vi "Data Read Multiple.vi"(0 "VISA resource name":refnum<visa-resource-name>, 1 "Source (0: Function)":u16(ring) items=["Function", "Calculation 1"], 2 "Format (0: ASCII)":u16(ring) items=["ASCII", "Single Precision", "Double Precision"], 3 "Number of Readings (100)":i32=100, 4 "Sample Count (1)":i32=1, 5 "error in (no error)":errorcluster, 8 "Timeout (25000 ms)":u32=25000) -> (14 "VISA resource name out":refnum<visa-resource-name>, 15 "Data":dbl[](array[numeric]), 16 "Channels":i32[](array[numeric]), 17 "Units":string[](array[string]), 19 "error out":errorcluster)   [LabVIEW 2016, in "Keithley 2000.lvlib"]
doc: "This VI reads multiple measurements or calculations from the instrument. This VI should be used instead of the Data Read Single VI when you plan on reading many measurements at once or when you are reading measurements from many channels."
uses:
  Keithley 2000.lvlib
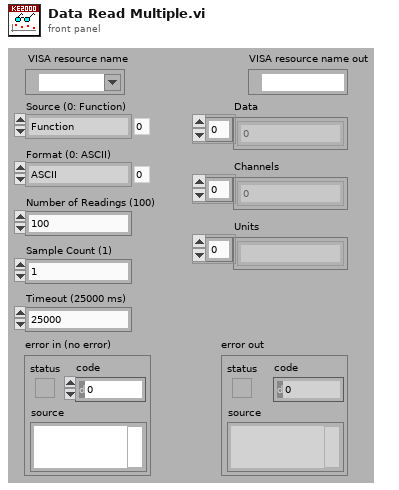
[diagram p1: front panel]
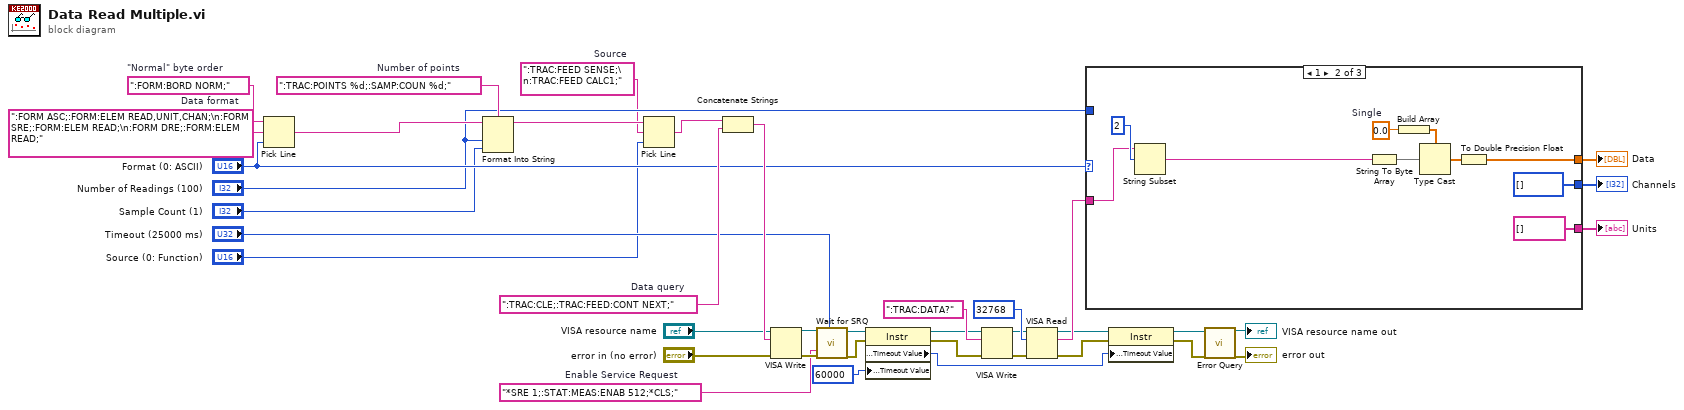
[diagram p0: block diagram]
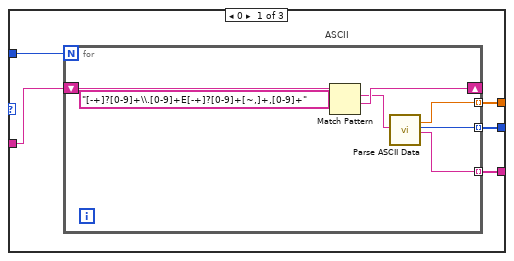
[diagram p2: hidden frame]
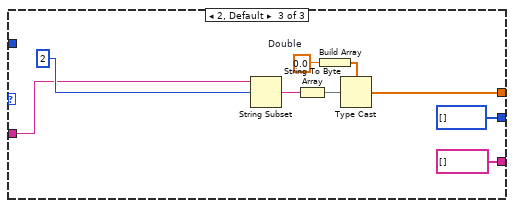
[diagram p3: hidden frame]
diagram:
  w19 = ":TRAC:FEED SENSE;\n:TRAC:FEED CALC1;"  # Source
  w1 = "*SRE 1;:STAT:MEAS:ENAB 512;*CLS;"  # Enable Service Request
  w36 = ":TRAC:POINTS %d;:SAMP:COUN %d;"  # Number of points
  w37 = ":FORM:BORD NORM;"  # "Normal" byte order
  w38 = ":FORM ASC;:FORM:ELEM READ,UNIT,CHAN;\n:FORM SRE;:FORM:ELEM READ;\n:FORM DRE;:FORM:ELEM READ;"  # Data format
  w34 = ":TRAC:CLE;:TRAC:FEED:CONT NEXT;"  # Data query
  n1 = Pick Line(string ("")=w37, multi-line string=w38, line index="Format (0: ASCII)") -> (output string=w35:string)
  n2 = Format Into String(format string=w36, initial string=w35, "Number of Readings (100)", "Sample Count (1)") -> (resulting string=w22:string)  [unwired: 1 in, 1 out]
  n3 = Pick Line(string ("")=w22, multi-line string=w19, line index="Source (0: Function)") -> (output string=w20:string)
  n4 = Concatenate Strings(w20, w34) -> (w33:string)
  n5 = VISA Write(VISA resource name="VISA resource name", write buffer=w33, error in (no error)="error in (no error)") -> (VISA resource name out=w28:refnum<visa-resource-name>, error out=w29:errorcluster)  [unwired: 1 out]
  n6 = call "Wait for SRQ.vi"("VISA resource name"=w28, "SRQ Enable Command"=w1, "error in (no error)"=w29, "Timeout (25000 ms)"="Timeout (25000 ms)") -> ("VISA resource name out"=w15:refnum<visa-resource-name>, "error out"=w14:errorcluster)  [unwired: 14 in]
  n7 = property class="Instr"(reference=w15, error in=w14, "General Settings:Timeout Value"=u32 60000) -> (reference out=w12:refnum<visa-resource-name>, error out=w11:errorcluster, "General Settings:Timeout Value"=w10:u32)
  n8 = VISA Write(VISA resource name=w12, write buffer=":TRAC:DATA?", error in (no error)=w11) -> (VISA resource name out=w17:refnum<visa-resource-name>, error out=w18:errorcluster)  [unwired: 1 out]
  n9 = VISA Read(VISA resource name=w17, byte count=u32 32768, error in (no error)=w18) -> (VISA resource name out=w9:refnum<visa-resource-name>, read buffer=w31:string, error out=w8:errorcluster)  [unwired: 1 out]
  n10 = case shown="1" "Format (0: ASCII)" {
    tunnel: [w43 w58 w64] -> w30
    tunnel: w31 -> [w44 w56 w66]
    tunnel: [w42 string[] [] string[] []] -> w26
    tunnel: [w41 i32[] [] i32[] []] -> w25
    tunnel: "Number of Readings (100)" -> [w40 _ _]
    frame 0 {
      # "ASCII"
      n11 = for {
        N: w40 -> [_]
        shift-right: [w50] -> _
        shift-left: w44 -> [w51]
        tunnel: [w47] -> w43 mode=indexing
        tunnel: [w46] -> w42 mode=indexing
        tunnel: [w45] -> w41 mode=indexing
        n12 = Match Pattern(string=w51, regular expression="[-+]?[0-9]+\\.[0-9]+E[-+]?[0-9]+[~,]+,[0-9]+") -> (match substring=w48:string, after substring=w50:string)  [unwired: 1 in, 2 out]
        n13 = call "Parse ASCII Data.vi"("ASCII Data (Empty)"=w48) -> ("Measurement"=w47:dbl, "Channel"=w45:i32, "Units"=w46:string)  [unwired: 16 in]
      }
    }
    frame 1 {
      w61 = sgl 0.0  # Single
      n14 = String Subset(string=w56, offset (0)=2) -> (substring=w55:string)  [unwired: 1 in]
      n15 = String To Byte Array(string=w55) -> (unsigned byte array=w59:u8[])
      n16 = Build Array(w61) -> (w60:sgl[])
      n17 = Type Cast(type=w60, x=w59) -> (*(type *) &x=w54:sgl[])
      n18 = To Double Precision Float(number=w54) -> (double precision float=w58:dbl[])
    }
    frame 2, Default {
      w70 = 0.0  # Double
      n19 = String Subset(string=w66, offset (0)=2) -> (substring=w65:string)  [unwired: 1 in]
      n20 = String To Byte Array(string=w65) -> (unsigned byte array=w68:u8[])
      n21 = Build Array(w70) -> (w69:dbl[])
      n22 = Type Cast(type=w69, x=w68) -> (*(type *) &x=w64:dbl[])
    }
  }
  "Data" <- w30
  "Channels" <- w25
  "Units" <- w26
  n23 = property class="Instr"(reference=w9, error in=w8, "General Settings:Timeout Value"=w10) -> (reference out=w7:refnum<visa-resource-name>, error out=w6:errorcluster)
  n24 = call "Error Query.vi"("VISA resource name"=w7, "error in (no error)"=w6) -> ("VISA resource name out"=→"VISA resource name out":refnum<visa-resource-name>, "error out"=→"error out":errorcluster)  [unwired: 14 in, 2 out]
